vi "List Buckets.vi"(8 "error in (no error)":errorcluster) -> (0 "error out":errorcluster, 3 "Buckets":T1[](array[typedef]))   [LabVIEW 2011, in "LV Interface for Amazon S3.lvlib"]
doc: "This operation <B>returns a list of all buckets owned by the authenticated sender</B> of the request. Anonymous requests cannot list buckets, and you cannot list buckets that you did not create."
uses:
  LV Interface for Amazon S3.lvlib
  Typedefs/AMZ_S3_API_Bucket.ctl
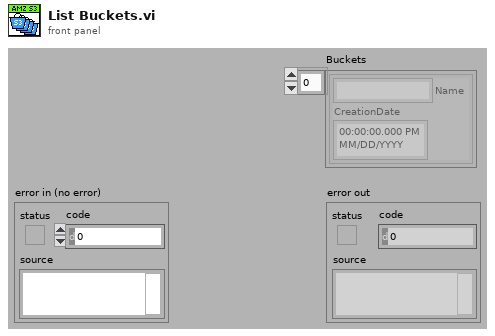
[diagram p1: front panel]
types:
  T1 = typedef "LV Interface for Amazon S3.lvlib/AMZ_S3_API_Bucket.ctl" = cluster{"Name":string, "CreationDate":timestamp}
  T2 = typedef "LV Interface for Amazon S3.lvlib/AMZ_S3_API_ListAllMyBucketsResult.ctl" = cluster{"Owner":T3, "Buckets":T1[]}
  T3 = typedef "LV Interface for Amazon S3.lvlib/AMZ_S3_API_Owner.ctl" = cluster{"ID":string, "DisplayName":string}
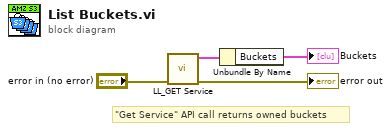
[diagram p0: block diagram]
diagram:
  # "\"Get Service\" API call returns owned buckets"
  n1 = call "LL_GET Service.vi"("error in (no error)"="error in (no error)") -> ("error out"=→"error out":errorcluster, "ListAllMyBucketsResult"=w2:T2)  [unwired: 8 in, 1 out]
  n2 = Unbundle By Name(w2) -> ("Buckets"=→"Buckets":T1[])
